vi "OEE_SCREEN_1_delete_pace_info.vi"(11 "cycle_time_and_pace":string[][](array[string])) -> ()   [LabVIEW 2019]
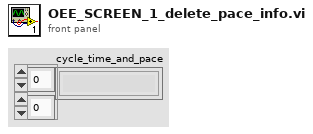
[diagram p1: front panel]
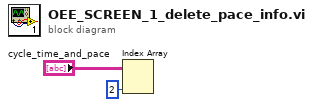
[diagram p0: block diagram]
diagram:
  n1 = Index Array(array="cycle_time_and_pace", index (col)=2 ("disabled index (col)")) -> ()  [unwired: 1 in, 1 out]
